vi "append_results_graph_bundle.vi"(1 "Y":cluster{dbl, dbl}[](array[cluster]), 2 "X":cluster{dbl, dbl}[](array[cluster])) -> (0 "concat(X,Y)":cluster{dbl, dbl}[](array[cluster]))   [LabVIEW 2017]
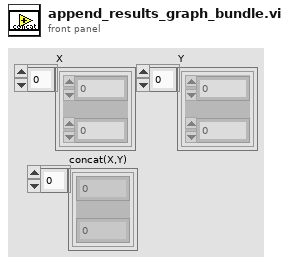
[diagram p1: front panel]
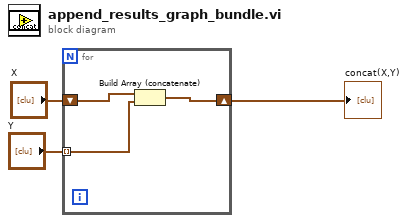
[diagram p0: block diagram]
diagram:
  n1 = for {
    tunnel: "Y" -> [w5] mode=indexing
    shift-right: [w4] -> w1
    shift-left: "X" -> [w6]
    n2 = Build Array (concatenate)(w6, w5) -> (w4:cluster{dbl, dbl}[])
  }
  "concat(X,Y)" <- w1
